vi "Insert Children.vi"(6 "Label Names":string[](array[string]), 7 "Metric Name":string, 8 "error in (no error)":errorcluster, 11 "Counter in":refnum<class "Counter.lvclass">) -> (0 "error out":errorcluster, 3 "Counter out":refnum<class "Counter.lvclass">)   [LabVIEW 2020, in "Metrics.lvlib" / "Counter.lvclass"]
uses:
  Counter.lvclass
  gauge/Gauge.lvclass
  C:/Github-locals/PromVIEW/src/metrics/metric/Metric.lvclass
  metric/Metric.lvclass/Metric.ctl
  Counter.lvclass/Counter.ctl
  metric/Write Name.vi
  metric/Write Label Names.vi
  metric/Validate Name.vi
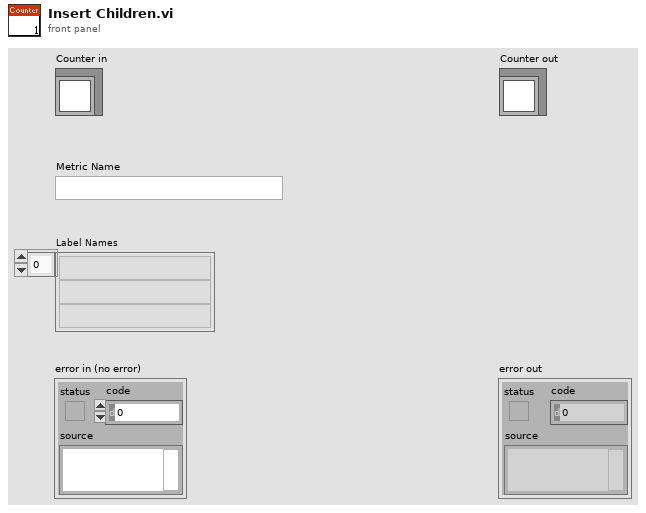
[diagram p1: front panel]
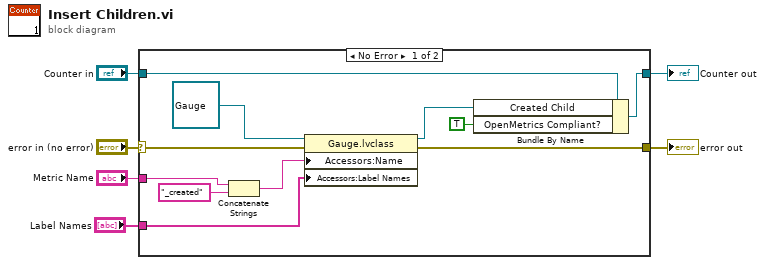
[diagram p0: block diagram]
diagram:
  n1 = case shown="No Error" "error in (no error)" {
    selector: "error in (no error)" -> [w10 w19]
    tunnel: [w9 w19] -> w5
    tunnel: [w16 w18] -> w3
    tunnel: "Counter in" -> [w17 w18]
    tunnel: "Metric Name" -> [w13 _]
    tunnel: "Label Names" -> [w7 _]
    frame No Error {
      n2 = Concatenate Strings(w13, "_created" ("string")) -> (w12:string)
      n3 = property class="Gauge.lvclass"(reference=refnum<class "Gauge.lvclass"> refnum ("Metrics.lvlib:Gauge.lvclass"), error in=w10, "Accessors:Name"=w12, "Accessors:Label Names"=w7) -> (reference out=w11:refnum<class "Gauge.lvclass">, error out=w9:errorcluster)
      n4 = Bundle By Name(cluster=w17, "Created Child"=w11, "OpenMetrics Compliant?"=TRUE) -> (w16:refnum<class "Counter.lvclass">)
    }
    frame Error {
    }
  }
  "error out" <- w5
  "Counter out" <- w3
